vi "ROS_Master_InventPID.vi"() -> (0 "XML":string)   [LabVIEW 2015]
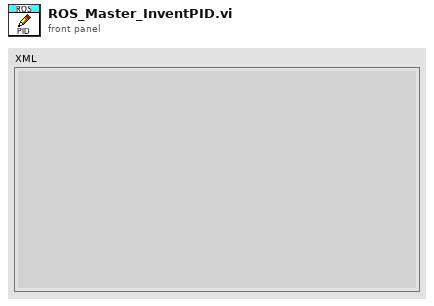
[diagram p1: front panel]
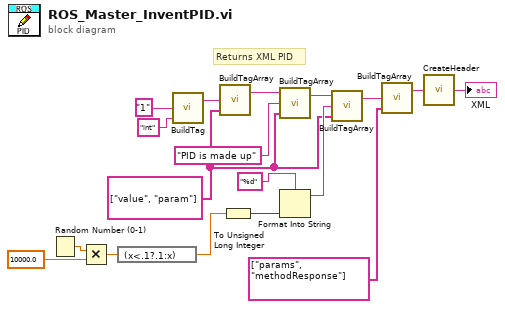
[diagram p0: block diagram]
diagram:
  w1 = string[] ["value", "param"] ("tags")
  # "Returns XML PID"
  n1 = Random Number (0-1)() -> (number: 0 to 1=w4:dbl)
  n2 = Multiply(x=w4, y=10000.0) -> (x*y=w13:dbl)
  n3 = expression code="(x<.1?.1:x)"(w13) -> (w14:dbl)
  n4 = call "BuildTag.vi"("tag"="int", "value"="1") -> ("string out"=w18:string)  [unwired: 2 in]
  n5 = call "BuildTagArray.vi"("tags"=w1, "value"=w18) -> ("string out"=w2:string)  [unwired: 2 in]
  n6 = To Unsigned Long Integer(number=w14) -> (unsigned 32bit integer=w6:u32)
  n7 = call "BuildTagArray.vi"("tags"=w1, "value"="PID is made up", "string in"=w2) -> ("string out"=w3:string)  [unwired: 1 in]
  n8 = Format Into String(format string="%d", w6) -> (resulting string=w8:string)  [unwired: 2 in, 1 out]
  n9 = call "BuildTagArray.vi"("tags"=w1, "value"=w8, "string in"=w3) -> ("string out"=w9:string)  [unwired: 1 in]
  n10 = call "BuildTagArray.vi"("tags"=string[] ["params", "methodResponse"], "value"=w9) -> ("string out"=w11:string)  [unwired: 2 in]
  n11 = call "CreateHeader.vi"("Content"=w11) -> ("XML"=→"XML":string)
